vi "SwitchesMirrors Test.vi"() -> ()   [LabVIEW 2014]
uses:
  support/Instrument Status.ctl
  SwitchesMirrors Refnum.ctl
  SwitchesMirrors Functions.ctl
  SwitchesMirrors Status.ctl
panel:
  out "Status":T1
  in  "Laser":bool
  in  "Video":bool
  in  "VISA Session":refnum<visa-resource-name>="COM10"
  in  "Delays (ms)":cluster{"Laser":u32, "Video":u32}={"Laser"=150, "Video"=950}
  in  "stop":bool
  # "LICENSED MATERIALS – PROPERTY OF IBM\nCopyright IBM Corp. 2016,\nALL RIGHTS RESERVED"
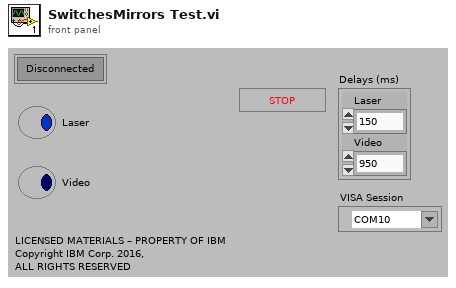
[diagram p1: front panel]
types:
  T1 = typedef "Instrument Status.ctl" = bool
  T2 = typedef "SwitchesMirrors Functions.ctl" = enum16{"Connect", "Get Configuration", "Set Configuration", "Update Refnums", "Disconnect"}
  T3 = typedef "SwitchesMirrors Refnum.ctl" = cluster{"Instrument Status":refnum<vi>, "Laser":refnum<vi>, "Video":refnum<vi>, "Relay VISA":refnum<vi>}
  T4 = typedef "SwitchesMirrors Status.ctl" = cluster{"Laser":bool, "Video":bool}
  T5 = enum32{"invalid app kind", "Development System", "Run Time System", "Student Edition", "Embedded LabVIEW", "Evaluation", "Custom"}
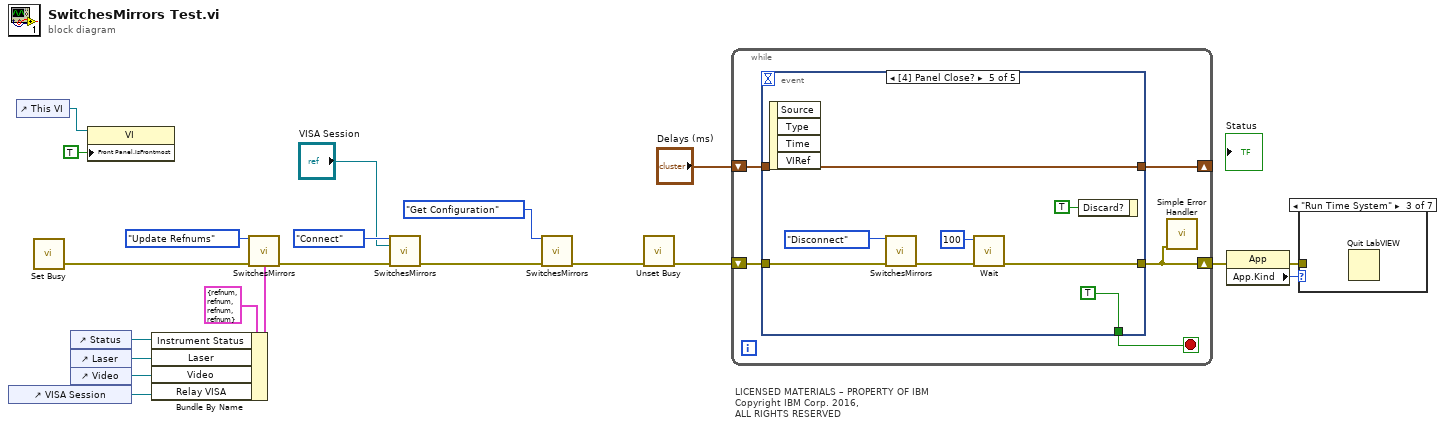
[diagram p0: block diagram]
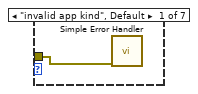
[diagram p2: hidden frame]
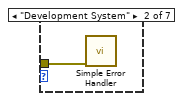
[diagram p3: hidden frame]
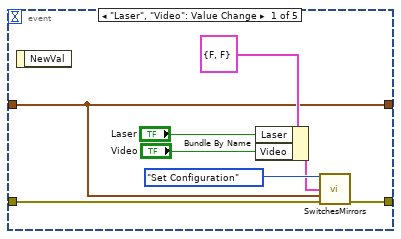
[diagram p8: hidden frame]
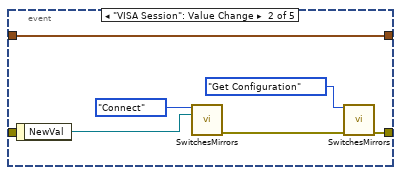
[diagram p9: hidden frame]
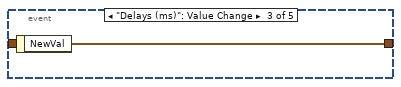
[diagram p10: hidden frame]
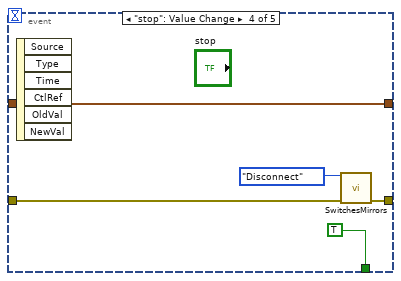
[diagram p11: hidden frame]
diagram:
  # "LICENSED MATERIALS – PROPERTY OF IBM\nCopyright IBM Corp. 2016,\nALL RIGHTS RESERVED"
  n1 = control-ref of="VISA Session"() -> (w15:refnum<vi>)
  n2 = control-ref of="This VI"() -> (w2:refnum<vi>)
  n3 = call <vilib>:"Set Busy.vi"() -> ("error out"=w4:errorcluster)  [unwired: 10 in, 1 out]
  n4 = control-ref of="Status"() -> (w19:refnum<vi>)
  n5 = control-ref of="Laser"() -> (w18:refnum<vi>)
  n6 = control-ref of="Video"() -> (w17:refnum<vi>)
  n7 = property class="VI"(reference=w2, "Front Panel.IsFrontmost"=TRUE ("Front Panel Window:Is Frontmost")) -> ()  [unwired: 1 in, 2 out]
  n8 = Bundle By Name(cluster=T3 {"Instrument Status"=refnum, "Laser"=refnum, "Video"=refnum, "Relay VISA"=refnum} ("Refnums"), "Instrument Status"=w19, "Laser"=w18, "Video"=w17, "Relay VISA"=w15) -> (w20:T3)
  n9 = call "SwitchesMirrors.vi"("Function"=SwitchesMirrors_Functions."Update Refnums", "Error In"=w4, "Refnums"=w20) -> ("Error Out"=w11:errorcluster)  [unwired: 11 in, 1 out]
  n10 = call "SwitchesMirrors.vi"("Function"=SwitchesMirrors_Functions."Connect", "Relay VISA Session"="VISA Session", "Error In"=w11) -> ("Error Out"=w13:errorcluster)  [unwired: 11 in, 1 out]
  n11 = call "SwitchesMirrors.vi"("Function"=SwitchesMirrors_Functions."Get Configuration", "Error In"=w13) -> ("Error Out"=w10:errorcluster)  [unwired: 12 in, 1 out]
  n12 = call <vilib>:"Unset Busy.vi"("error in (no error)"=w10) -> ("error out"=w3:errorcluster)  [unwired: 10 in]
  n13 = while {
    shift-right: [w23] -> _
    shift-left: "Delays (ms)" -> [w22]
    shift-right: [w24] -> w5
    shift-left: w3 -> [w26]
    stop <- w25 stop-if-true
    n14 = event shown="[4] Panel Close?" {
      selector: _ -> [_ _ _ _ _]
      dyn-events: _ -> [_ _ _ _ _]
      timeout: _ -> [_ _ _ _ _]
      tunnel: [w32 w37 _ w44 w48] -> w24
      tunnel: w26 -> [w33 _ _ w42 w50]
      tunnel: [_ _ _ TRUE TRUE] -> w25
      tunnel: [w27 w35 w41 w43 w51] -> w23
      tunnel: w22 -> [w27 w35 _ w43 w51]
      event "Laser", "Video": Value Change {
        n15 = event-data() -> ()  [unwired: 1 in, 1 out]
        n16 = Bundle By Name(cluster=T4 {"Laser"=FALSE, "Video"=FALSE} ("Set Switch"), "Laser"="Laser", "Video"="Video") -> (w30:T4)
        n17 = call "SwitchesMirrors.vi"("Function"=SwitchesMirrors_Functions."Set Configuration", "Set Switch"=w30, "Delays (ms)"=w27, "Error In"=w33) -> ("Error Out"=w32:errorcluster)  [unwired: 10 in, 1 out]
      }
      event "VISA Session": Value Change {
        n18 = event-data() -> ("NewVal"=w36:refnum<visa-resource-name>)  [unwired: 1 in]
        n19 = call "SwitchesMirrors.vi"("Function"=SwitchesMirrors_Functions."Connect", "Relay VISA Session"=w36) -> ("Error Out"=w39:errorcluster)  [unwired: 12 in, 1 out]
        n20 = call "SwitchesMirrors.vi"("Function"=SwitchesMirrors_Functions."Get Configuration", "Error In"=w39) -> ("Error Out"=w37:errorcluster)  [unwired: 12 in, 1 out]
      }
      event "Delays (ms)": Value Change {
        n21 = event-data() -> ("NewVal"=w41:cluster{"Laser":u32, "Video":u32})  [unwired: 1 in]
      }
      event "stop": Value Change {
        n22 = event-data() -> ()  [unwired: 1 in, 6 out]
        n23 = call "SwitchesMirrors.vi"("Function"=SwitchesMirrors_Functions."Disconnect", "Error In"=w42) -> ("Error Out"=w44:errorcluster)  [unwired: 12 in, 1 out]
      }
      event Panel Close? {
        n24 = event-data() -> ()  [unwired: 1 in, 4 out]
        n25 = call "SwitchesMirrors.vi"("Function"=SwitchesMirrors_Functions."Disconnect", "Error In"=w50) -> ("Error Out"=w52:errorcluster)  [unwired: 12 in, 1 out]
        n26 = call "Wait.vi"("error in (no error)"=w52, "milliseconds to wait"=u32 100) -> ("error out"=w48:errorcluster)  [unwired: 9 in]
        n27 = event-data("Discard?"=TRUE) -> ()  [unwired: 1 in, 1 out]
      }
    }
    n28 = call <vilib>:"Simple Error Handler.vi"("error in (no error)"=w24) -> ()  [unwired: 4 in, 5 out]
  }
  n29 = property class="App"(error in=w5) -> (error out=w6:errorcluster, "App.Kind"=w7:T5)  [unwired: 1 in, 1 out]
  n30 = case shown="\"Run Time System\"" w7 {
    tunnel: w6 -> [w55 w56 _ _ _ _ _]
    frame "invalid app kind", Default {
      n31 = call <vilib>:"Simple Error Handler.vi"("error in (no error)"=w55) -> ()  [unwired: 1 in, 8 out]
    }
    frame "Development System" {
      n32 = call <vilib>:"Simple Error Handler.vi"("error in (no error)"=w56) -> ()  [unwired: 1 in, 8 out]
    }
    frame "Run Time System" {
      n33 = Quit LabVIEW() -> ()  [unwired: 1 out]
    }
    frame "Student Edition" {
    }
    frame "Embedded LabVIEW" {
    }
    frame "Evaluation" {
    }
    frame "Custom" {
    }
  }
